vi "布尔切换型入队.vi"(8 "字符串":string, 9 "true启用入队":bool, 10 "控件引用":refnum<vi>, 11 "消息入队列":refnum<queue>) -> ()   [LabVIEW 2018]
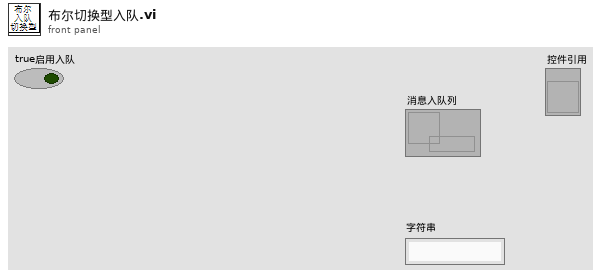
[diagram p1: front panel]
types:
  T1 = enum8{"Enabled", "Disabled", "Disabled and Grayed Out"}
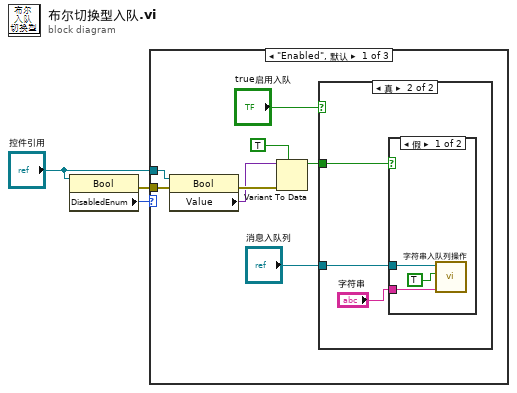
[diagram p0: block diagram]
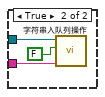
[diagram p3: hidden frame]
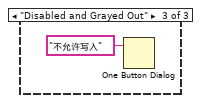
[diagram p5: hidden frame]
diagram:
  n1 = property class="Bool"(reference="控件引用") -> (error out=w1:errorcluster, "DisabledEnum"=w3:T1)  [unwired: 1 in, 1 out]
  n2 = case shown="\"Enabled\", 默认" w3 {
    tunnel: "控件引用" -> [w8 _ _]
    tunnel: w1 -> [w4 _ _]
    frame "Enabled", Default {
      n3 = property class="Bool"(reference=w8, error in=w4) -> (error out=w11:errorcluster, "Value"=w10:variant)  [unwired: 1 out]
      n4 = Variant To Data(error in=w11, type=TRUE, Variant=w10) -> (data=w6:bool)  [unwired: 1 out]
      n5 = case shown="真" "true启用入队" {
        tunnel: "消息入队列" -> [_ w13]
        tunnel: w6 -> [_ w12]
        frame False {
        }
        frame True {
          n6 = case shown="假" w12 {
            tunnel: w13 -> [w17 w20]
            tunnel: "字符串" -> [w16 w19]
            frame False {
              n7 = call "字符串入队列操作.vi"("字符消息入队列"=w16, "布尔"=TRUE, "界面切换队列"=w17) -> ()  [unwired: 8 in, 1 out]
            }
            frame True {
              n8 = call "字符串入队列操作.vi"("字符消息入队列"=w19, "布尔"=FALSE, "界面切换队列"=w20) -> ()  [unwired: 8 in, 1 out]
            }
          }
        }
      }
    }
    frame "Disabled" {
    }
    frame "Disabled and Grayed Out" {
      n9 = One Button Dialog(message="不允许写入" ("消息")) -> ()  [unwired: 1 in, 1 out]
    }
  }
